vi "Tones Measurement.vi"(8 "error in":errorcluster, 11 "wfm":waveform(dbl)) -> (0 "error out":errorcluster, 2 "Detected Amplitudes":dbl[](array[numeric]) format="%_2g", 3 "Detected Frequencies":dbl[](array[numeric]) format="%#_2p")   [LabVIEW 2024, in "NIScopeFrequencyDomain.lvlib"]
uses:
  NIScopeFrequencyDomain.lvlib
  <vilib>/measure/matone.llb/Extract Multiple Tone Information 1 Chan.vi
  <vilib>/measure/NI_MAPro.lvlib
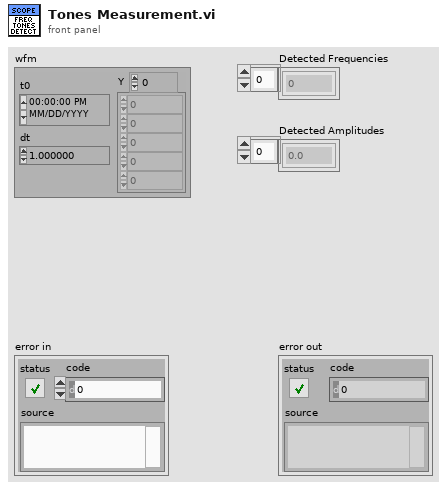
[diagram p1: front panel]
types:
  T1 = cluster{"detected frequency":dbl, "detected amplitude":dbl, "detected phase (deg)":dbl}[]
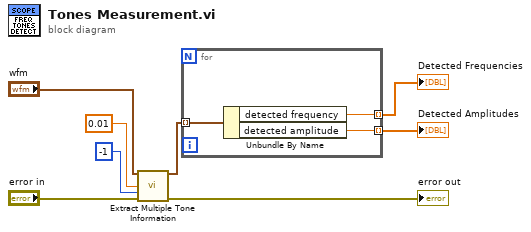
[diagram p0: block diagram]
diagram:
  n1 = call-poly <vilib>:"Extract Multiple Tone Information.vi"("time signal in"="wfm", "threshold"=0.01, "max num tones"=-1, "error in (no error)"="error in") -> ("multiple tone information"=w6:T1, "error out"=→"error out":errorcluster)  [unwired: 9 in, 1 out]
  n2 = for {
    tunnel: w6 -> [w11] mode=indexing
    tunnel: [w10] -> w7 mode=indexing
    tunnel: [w9] -> w8 mode=indexing
    n3 = Unbundle By Name(w11) -> ("detected frequency"=w10:dbl, "detected amplitude"=w9:dbl)
  }
  "Detected Amplitudes" <- w8
  "Detected Frequencies" <- w7
